vi "collate 3d data.vi"(10 "sorted input data":cluster{"type":dbl, "time":dbl, "data":dbl}[](array[cluster]), 11 "leftover":cluster{"type":dbl, "time":dbl, "data":dbl}[](array[cluster])) -> (2 "3d vs t data":T1[](array[typedef]), 3 "leftover to feedback":cluster{"type":dbl, "time":dbl, "data":dbl}[](array[cluster]))   [LabVIEW 2017]
uses:
  typedefs/reading3.ctl
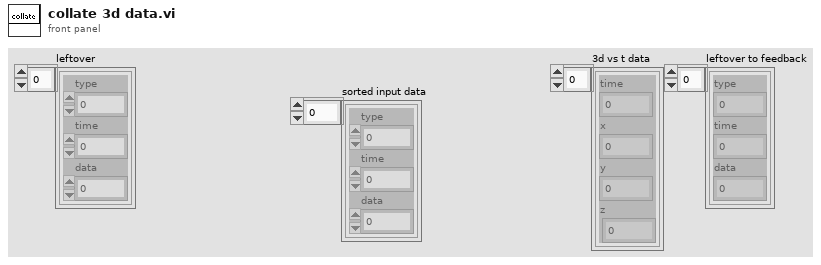
[diagram p1: front panel]
types:
  T1 = typedef "reading3.ctl" = cluster{"time":dbl, "x":dbl, "y":dbl, "z":dbl}
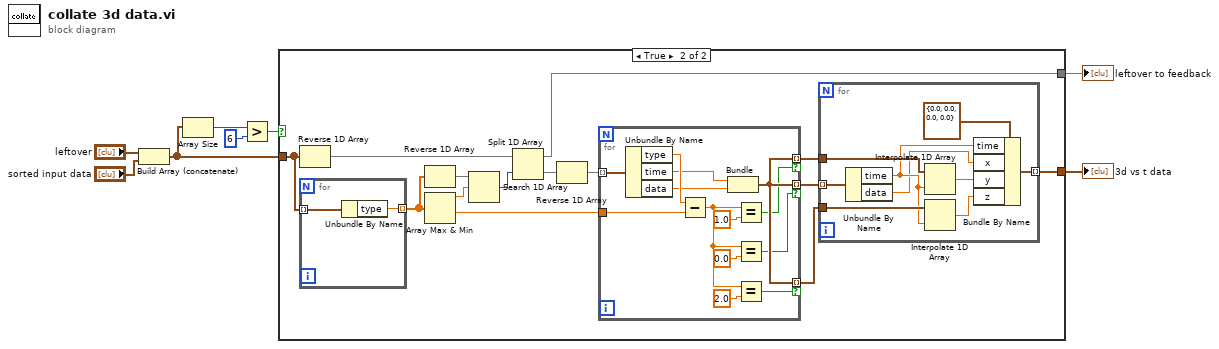
[diagram p0: block diagram]
diagram:
  n1 = Build Array (concatenate)("leftover", "sorted input data") -> (w5:cluster{"type":dbl, "time":dbl, "data":dbl}[])
  n2 = Array Size(array=w5) -> (size(s)=w4:i32)
  n3 = Greater?(x=w4, y=6) -> (0:w2:bool)
  n4 = case shown="True" w2 {
    tunnel: [_ w20] -> w7
    tunnel: w5 -> [w9 w11]
    tunnel: [w9 w10] -> w1
    frame False {
    }
    frame True {
      n5 = Reverse 1D Array(array=w11) -> (reversed array=w16:cluster{"type":dbl, "time":dbl, "data":dbl}[])
      n6 = for {
        tunnel: w11 -> [w47] mode=indexing
        tunnel: [w46] -> w19 mode=indexing
        n7 = Unbundle By Name(w47) -> ("type"=w46:dbl)
      }
      n8 = Reverse 1D Array(array=w19) -> (reversed array=w18:dbl[])
      n9 = Array Max & Min(array=w19) -> (max value=w14:dbl, min value=w17:dbl)  [unwired: 2 out]
      n10 = Search 1D Array(1D array=w18, element=w14) -> (index of element=w13:i32)  [unwired: 1 in]
      n11 = Split 1D Array(array=w16, index=w13) -> (first subarray=w10:cluster{"type":dbl, "time":dbl, "data":dbl}[], second subarray=w15:cluster{"type":dbl, "time":dbl, "data":dbl}[])
      n12 = Reverse 1D Array(array=w15) -> (reversed array=w12:cluster{"type":dbl, "time":dbl, "data":dbl}[])
      n13 = for {
        tunnel: w12 -> [w45] mode=indexing
        tunnel: w17 -> [w43]
        tunnel: [w36] -> w22 mode=indexing if=w35
        tunnel: [w36] -> w23 mode=indexing if=w34
        tunnel: [w36] -> w21 mode=indexing if=w33
        n14 = Unbundle By Name(w45) -> ("type"=w44:dbl, "time"=w38:dbl, "data"=w37:dbl)
        n15 = Subtract(x=w44, y=w43) -> (x-y=w39:dbl)
        n16 = Bundle("time"=w38, "data"=w37) -> (w36:cluster{"time":dbl, "data":dbl})  [unwired: 1 in]
        n17 = Equal?(x=w39, y=1.0) -> (x = y?=w34:bool)
        n18 = Equal?(x=w39, y=0.0) -> (x = y?=w35:bool)
        n19 = Equal?(x=w39, y=2.0) -> (x = y?=w33:bool)
      }
      n20 = for {
        tunnel: w23 -> [w32]
        tunnel: w22 -> [w31] mode=indexing
        tunnel: w21 -> [w30]
        tunnel: [w24] -> w20 mode=indexing
        n21 = Unbundle By Name(w31) -> ("time"=w28:dbl, "data"=w26:dbl)
        n22 = Interpolate 1D Array(1:w28, 2:w32) -> (0:w27:dbl)
        n23 = Interpolate 1D Array(1:w28, 2:w30) -> (0:w25:dbl)
        n24 = Bundle By Name(cluster=T1 {"time"=0.0, "x"=0.0, "y"=0.0, "z"=0.0} ("reading3"), "time"=w28, "x"=w26, "y"=w27, "z"=w25) -> (w24:T1)
      }
    }
  }
  "3d vs t data" <- w7
  "leftover to feedback" <- w1
